vi "speed set (SubVI).vi"(3 "speed(r/min)":i32, 4 "보내기":T1={"국번"="0", "커맨드"="A0", "데이터 No."="10"}, 5 "VISA 참조 번호 입력":refnum<visa-resource-name>) -> (0 "x = y?":bool, 2 "VISA 참조 번호 출력":refnum<visa-resource-name>)   [LabVIEW 2014]
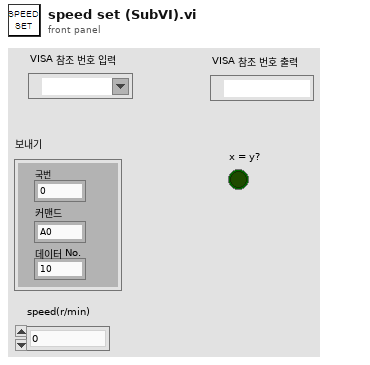
[diagram p1: front panel]
types:
  T1 = cluster{"국번":string, "커맨드":string, "데이터 No.":string}
  T2 = cluster{"국번":string, "커맨드":string, "데이터 No.":string, string}
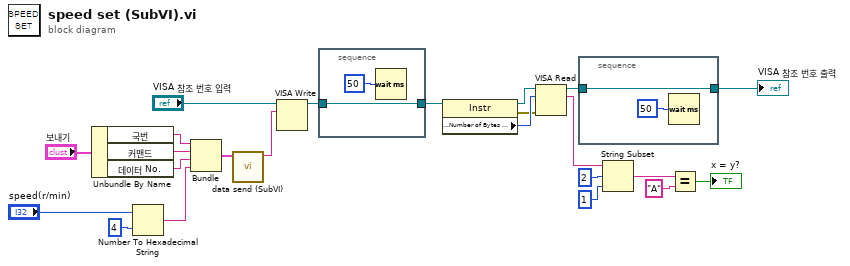
[diagram p0: block diagram]
diagram:
  n1 = Unbundle By Name("보내기") -> ("국번"=w20:string, "커맨드"=w19:string, "데이터 No."=w18:string)
  n2 = Number To Hexadecimal String(1:i16 4 ("폭(-)"), 2:"speed(r/min)") -> (0:w17:string)
  n3 = Bundle("국번"=w20, "커맨드"=w19, "데이터 No."=w18, w17) -> (w1:T2)  [unwired: 1 in]
  n4 = call "data send (SubVI).vi"("보내기"=w1) -> ("문자열"=w4:string)  [unwired: 10 in]
  n5 = VISA Write(VISA resource name="VISA 참조 번호 입력", write buffer=w4) -> (VISA resource name out=w10:refnum<visa-resource-name>)  [unwired: 1 in, 2 out]
  n6 = stacked-sequence {
    tunnel: w10 -> [w25]
    tunnel: [w25] -> w6
    frame #0 {
      n7 = Wait (ms)(milliseconds to wait=u32 50 ("delay before read (ms)")) -> ()  [unwired: 1 out]
    }
  }
  n8 = property on="Property Node" class="Instr"(reference=w6) -> (reference out=w7:refnum<visa-resource-name>, error out=w8:errorcluster, "Serial Settings:Number of Bytes at Serial Port"=w9:u32)  [unwired: 1 in]
  n9 = VISA Read(VISA resource name=w7, byte count=w9, error in (no error)=w8) -> (VISA resource name out=w3:refnum<visa-resource-name>, read buffer=w13:string)  [unwired: 2 out]
  n10 = stacked-sequence {
    tunnel: w3 -> [w27]
    tunnel: [w27] -> w2
    frame #0 {
      n11 = Wait (ms)(milliseconds to wait=u32 50 ("delay before read (ms)")) -> ()  [unwired: 1 out]
    }
  }
  "VISA 참조 번호 출력" <- w2
  n12 = String Subset(string=w13, offset (0)=2 ("오프셋(0)"), length (rest)=1 ("길이(나머지)")) -> (substring=w14:string)
  n13 = Equal?(x=w14, y="A") -> (x = y?=→"x = y?":bool)
